vi "Config Pulse V Measure I Sweep.vi"(0 "VISA resource name":refnum<visa-resource-name>, 1 "Channel (Channel A)":T1, 2 "Points (1)":u32=1 min=1, 3 "Tag (1)":u32=1 min=1, 4 "Buffer (nil)":string="nil", 7 "error in":errorcluster, 8 "Bias (0)":dbl, 9 "Sync In":u32, 10 "Start":dbl=1.0, 11 "Sync Out":u32, 12 "Stop":dbl=1.0, 13 "Sync In Timeout (10e-3)":dbl, 14 "Limit":dbl=0.001, 15 "Sync In Abort (True)":bool=TRUE, 16 "On Time":dbl=0.001, 18 "Off Time":dbl=0.001) -> (19 "Command String":string, 20 "VISA resource name out":refnum<visa-resource-name>, 22 "Success":bool, 25 "Message":string, 27 "error out":errorcluster)   [LabVIEW 2009, in "Keithley 2600 Series.lvlib"]
doc: "This VI configures a voltage pulse sweep using the KIFactoryPulse Script.\n\n<b>Functions and Attributes Used</b>\nConfigPulseVMeasureISweepLin()\nConfigPulseVMeasureISweepLog()"
uses:
  <instrlib>/Keithley 2600 Series/Keithley 2600 Series.lvlib
  <instrlib>/Keithley 2600 Series/Public/Channel.ctl
  <instrlib>/Keithley 2600 Series/Private/GlobalVariables.vi
panel:
  in  "Sweep Type":enum16{"Linear", "Logarithmic"}(ring)
  # "(c) 2008 Keithley Instruments, Inc.  ALL RIGHTS RESERVED."
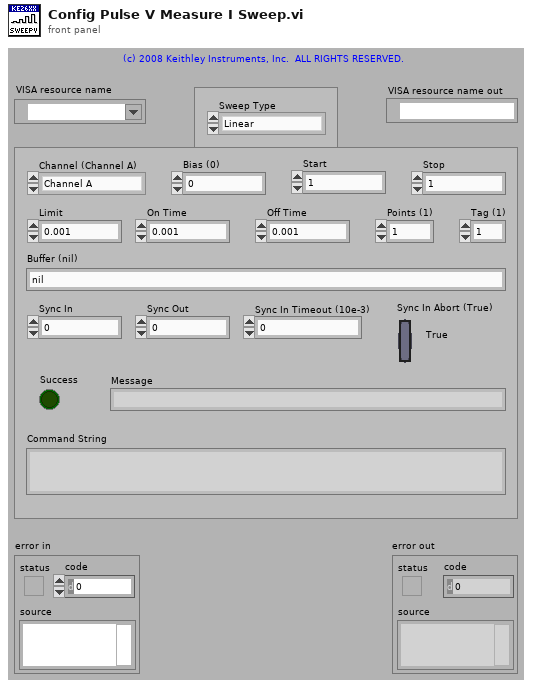
[diagram p1: front panel]
types:
  T1 = typedef "Keithley 2600 Series.lvlib/Channel.ctl" = enum32{"Channel A", "Channel B"}
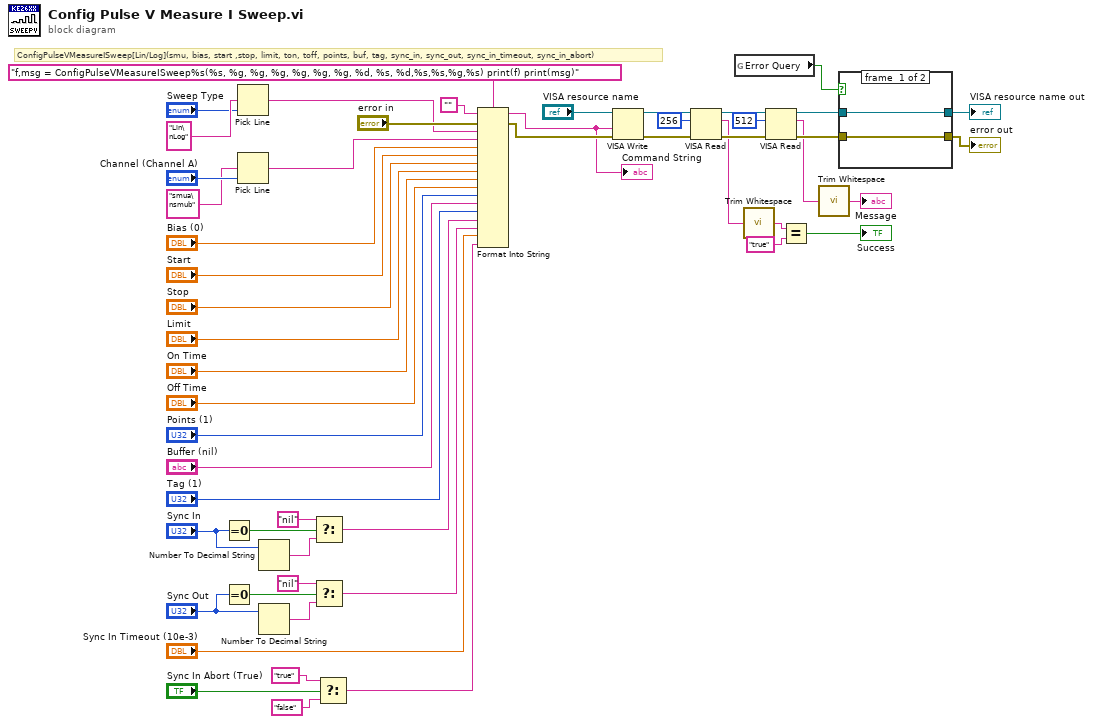
[diagram p0: block diagram]
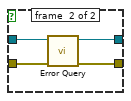
[diagram p2: hidden frame]
diagram:
  # "ConfigPulseVMeasureISweep[Lin/Log](smu, bias, start ,stop, limit, ton, toff, points, buf, tag, sync_in, sync_out, sync_in_timeout, sync_in_abort)"
  n1 = Equal To 0?(x="Sync In") -> (x = 0?=w26:bool)
  n2 = Equal To 0?(x="Sync Out") -> (x = 0?=w23:bool)
  n3 = Pick Line(multi-line string="Lin\nLog", line index="Sweep Type") -> (output string=w1:string)  [unwired: 1 out]
  n4 = Pick Line(multi-line string="smua\nsmub", line index="Channel (Channel A)") -> (output string=w2:string)  [unwired: 1 out]
  n5 = Number To Decimal String(number="Sync In") -> (decimal integer string=w24:string)  [unwired: 1 out]
  n6 = Number To Decimal String(number="Sync Out") -> (decimal integer string=w21:string)  [unwired: 1 out]
  n7 = Select(t="nil", s=w26, f=w24) -> (s? t:f=w12:string)
  n8 = Select(t="nil", s=w23, f=w21) -> (s? t:f=w13:string)
  n9 = Select(t="true", s="Sync In Abort (True)", f="false") -> (s? t:f=w15:string)
  n10 = Format Into String(format string="f,msg = ConfigPulseVMeasureISweep%s(%s, %g, %g, %g, %g, %g, %g, %d, %s, %d,%s,%s,%g,%s) print(f) print(msg)", initial string="", error in="error in", w1, w2, "Bias (0)", "Start", "Stop", "Limit", "On Time", "Off Time", "Points (1)", "Buffer (nil)", "Tag (1)", w12, w13, "Sync In Timeout (10e-3)", w15) -> (resulting string=w33:string, error out=w51:errorcluster)
  "Command String" <- w33
  n11 = VISA Write(VISA resource name="VISA resource name", write buffer=w33, error in (no error)=w51) -> (VISA resource name out=w49:refnum<visa-resource-name>, error out=w50:errorcluster)  [unwired: 1 out]
  n12 = VISA Read(VISA resource name=w49, byte count=u32 256, error in (no error)=w50) -> (VISA resource name out=w48:refnum<visa-resource-name>, read buffer=w46:string, error out=w47:errorcluster)  [unwired: 1 out]
  n13 = global read "GlobalVariables.vi" "Error Query"() -> (w43:bool)
  n14 = call <vilib>:"Trim Whitespace.vi"("string"=w46) -> ("trimmed string"=w45:string)  [unwired: 1 in]
  n15 = VISA Read(VISA resource name=w48, byte count=u32 512, error in (no error)=w47) -> (VISA resource name out=w41:refnum<visa-resource-name>, read buffer=w34:string, error out=w42:errorcluster)  [unwired: 1 out]
  n16 = Equal?(x=w45, y="true") -> (x = y?=→"Success":bool)
  n17 = call <vilib>:"Trim Whitespace.vi"("string"=w34) -> ("trimmed string"=→"Message":string)  [unwired: 1 in]
  n18 = case shown="True" w43 {
    tunnel: w41 -> [w55 w59]
    tunnel: w42 -> [w54 w58]
    tunnel: [w55 w57] -> w38
    tunnel: [w54 w56] -> w37
    frame #0 {
    }
    frame #1 {
      n19 = call <instrlib>:"Error Query.vi"("error in (no error)"=w58, "VISA resource name"=w59) -> ("error out"=w56:errorcluster, "VISA resource name out"=w57:refnum<visa-resource-name>)  [unwired: 8 out]
    }
  }
  "VISA resource name out" <- w38
  "error out" <- w37
